vi "FrontPanel.vi"() -> ()   [LabVIEW 2017, in "ImageAcquisitionLibrary.lvlib"]
uses:
  ImageAcquisitionLibrary.lvlib
  StopButton.ctl
  QueueOperations/Message Cluster.ctl
  Acquisition/AcquisitionLoopState.ctl
  Tracking/Tracking State.ctl
  Recording/RecordingState.ctl
  Acquisition/AcquireData.ctl
  MarkersArray.ctl
  Marker.ctl
  <vilib>/Utility/error.llb/DialogType.ctl
  ImageNotifier.vi
  QueueOperations/Enqueue Message (Single).vi
  GlobalFrontPanelReferences.vi
  SettingsGlobal.vi
  MessageQueue.lvlib
panel:
  out "Tracking":i32
  out "Dropped":u32
  out "Image":i32
  in  "Stop":T1
  in  "Settings":bool
  in  "Tracking":bool
  in  "Acquire":bool
  in  "Rec":bool
  out "Image":T2(plugin-control)
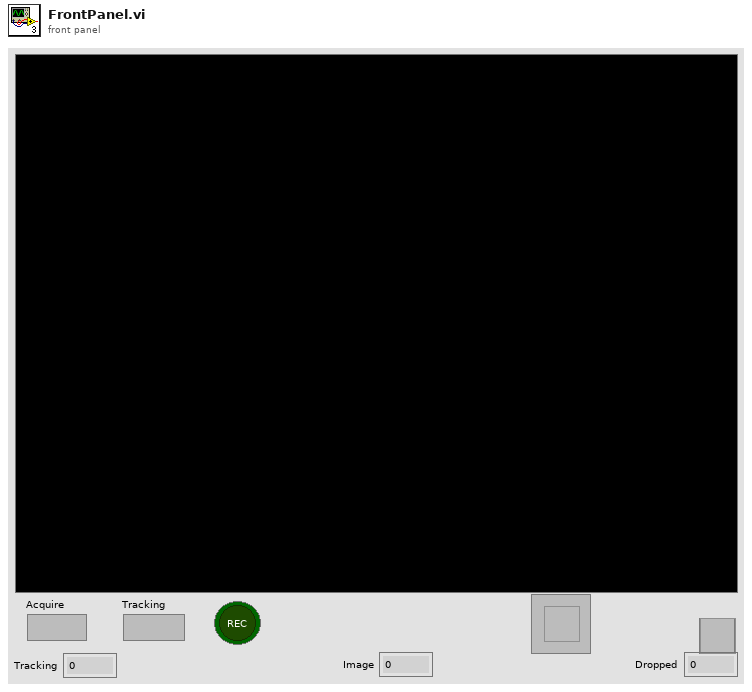
[diagram p1: front panel]
types:
  T1 = typedef "ImageAcquisitionLibrary.lvlib/StopButton.ctl" = bool
  T2 = typedef "IMAQ Image.ctl" = refnum<image>
  T3 = typedef "Image Type" = u32
  T4 = typedef "ImageAcquisitionLibrary.lvlib/AcquireData.ctl" = cluster{"Frame Data":cluster{"Image":u32[][], "Timestamp":timestamp, "Image Type":T3, "Dropped Frames":u32}, "Tracking Data":cluster{"Positions":dbl[][], "Timestamp":timestamp}, "Tracked?":bool}
  T5 = typedef "ImageAcquisitionLibrary.lvlib/RecordingState.ctl" = enum16{"Idle", "Start Recording", "Record", "Update Settings", "Stop Recording", "Exit"}
  T6 = typedef "ImageAcquisitionLibrary.lvlib/Tracking State.ctl" = enum16{"Idle", "Start Tracking", "Track", "Stop Tracking", "Update Settings", "Exit"}
  T7 = typedef "ImageAcquisitionLibrary.lvlib/AcquisitionLoopState.ctl" = enum16{"Start Acquisition", "Acquire", "Stop Acquisition", "Update Settings", "Exit"}
  T8 = typedef "ImageAcquisitionLibrary.lvlib/MessageQueue.lvlib/Message Cluster.ctl" = cluster{"Message":string, "Message Data":variant}
  T9 = typedef "ImageAcquisitionLibrary.lvlib/References.ctl" = cluster{"Acquire":refnum<vi>, "Rec":refnum<vi>, "Tracking":refnum<vi>, "Settings":refnum<vi>, "Stop":refnum<vi>, "Initialized?":bool, "ImDisplay":refnum<vi>}
  T10 = typedef "ImageAcquisitionLibrary.lvlib/Settings.ctl" = cluster{"Harware Configuration":cluster{"Camera":T11, "Frames Per Second":u32, "Simulate Recording":bool, "Simulated Recording Sample":path, "Timestamp Method":enum16{"System Timestamp", "Camera Timestamp", "IMAQdx Timestamp"}}, "Base Recording Path":path, "Type Of Recording":string, "Recording Codec":string, "TrackingSettings":T12, "Calibration":T14, "Broadcast Length":i32}
  T11 = typedef "IMAQdx.ctl" = refnum<k21>
  T12 = typedef "ImageAcquisitionLibrary.lvlib/TrackingSettings.ctl" = cluster{"Max Radius":i32, "Threshold":sgl, "ROI":T13}
  T13 = typedef "IMAQ Rectangle" = cluster{"Left":i32, "Top":i32, "Right":i32, "Bottom":i32, "Rotation":dbl}
  T14 = typedef "ImageAcquisitionLibrary.lvlib/Calibration.ctl" = cluster{"Pixel Width (X)":dbl, "Pixel Height (Y)":dbl}
  T15 = typedef "ImageAcquisitionLibrary.lvlib/MarkersArray.ctl" = T16[]
  T16 = typedef "ImageAcquisitionLibrary.lvlib/Marker.ctl" = cluster{"X":dbl, "Color":u32, "Y ":dbl, "Owner":u8}
  T17 = typedef "DialogType.ctl" = u16
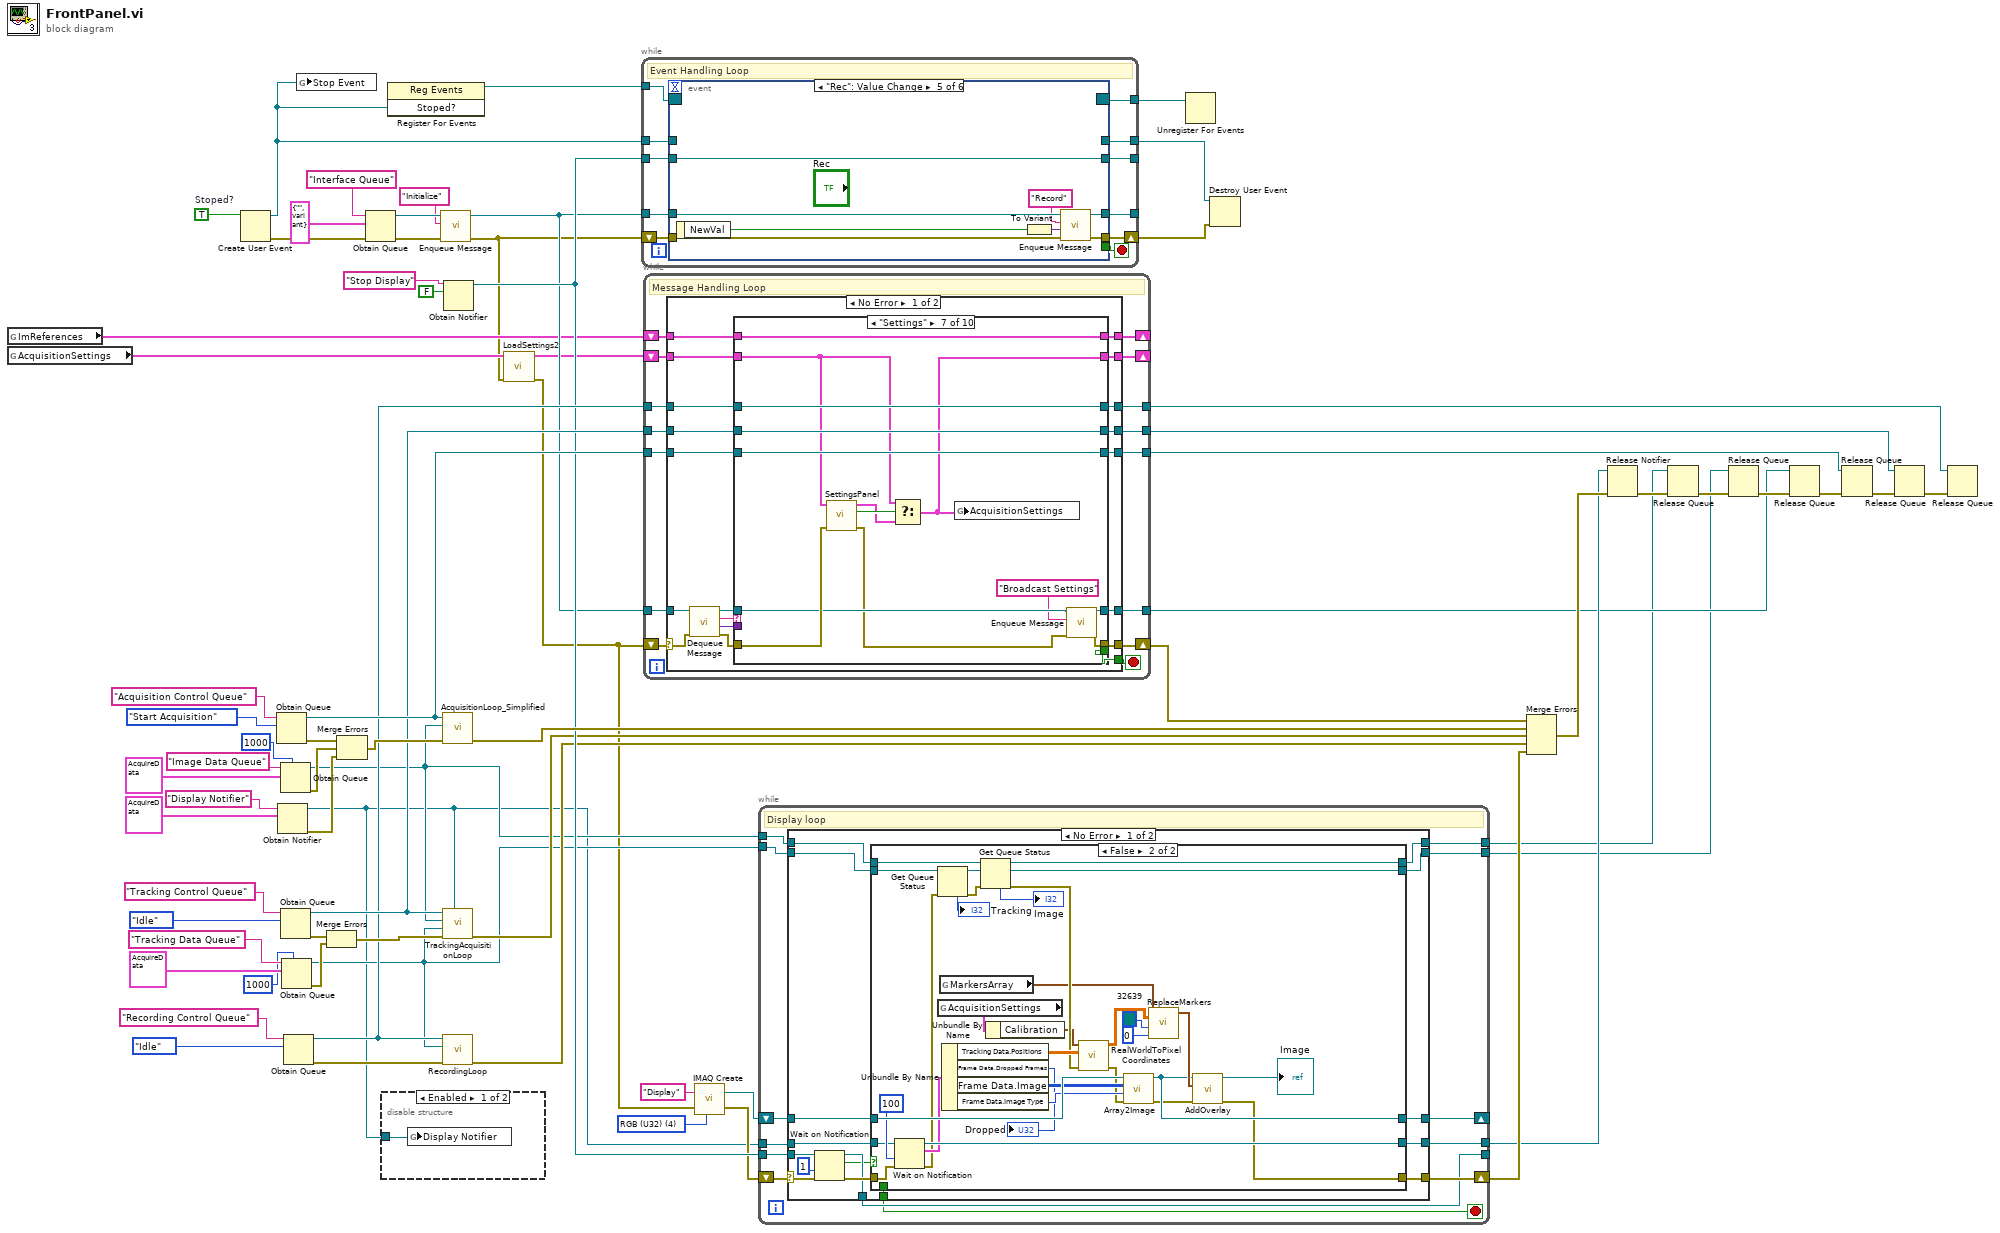
[diagram p0: block diagram]
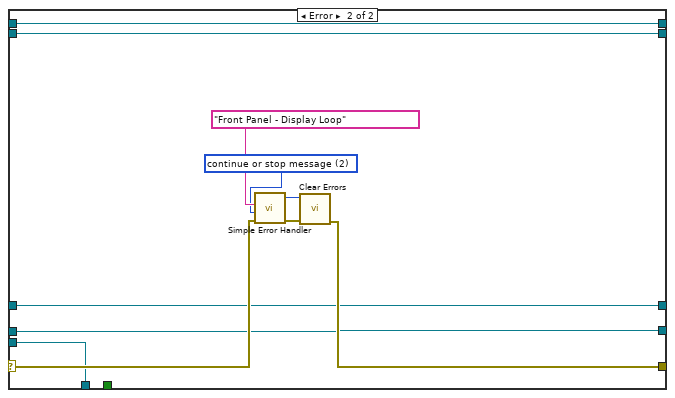
[diagram p4: hidden frame]
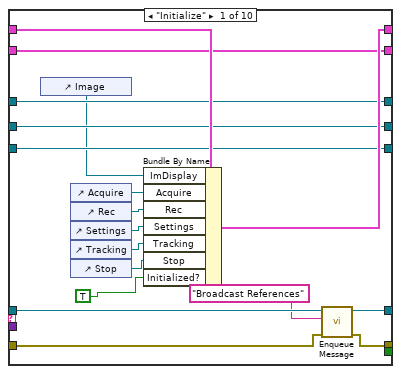
[diagram p5: hidden frame]
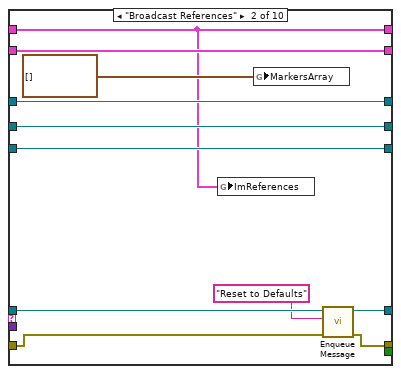
[diagram p6: hidden frame]
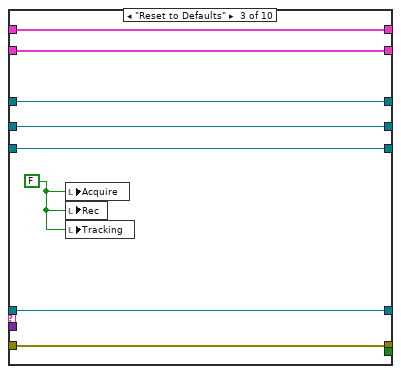
[diagram p7: hidden frame]
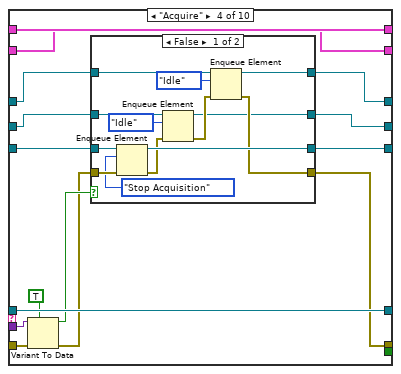
[diagram p8: hidden frame]
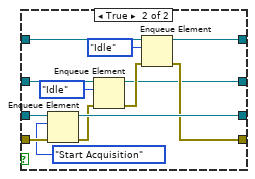
[diagram p9: hidden frame]
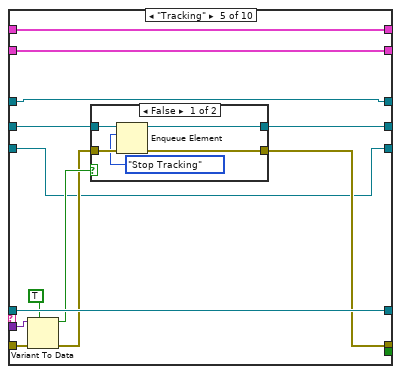
[diagram p10: hidden frame]
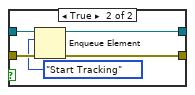
[diagram p11: hidden frame]
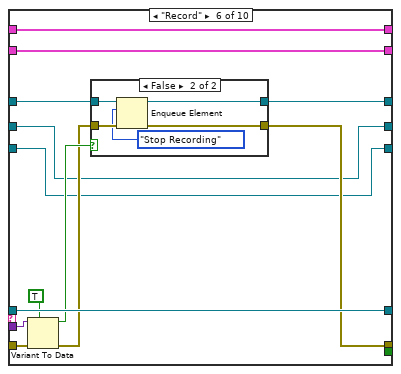
[diagram p12: hidden frame]
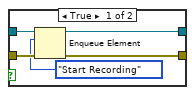
[diagram p13: hidden frame]
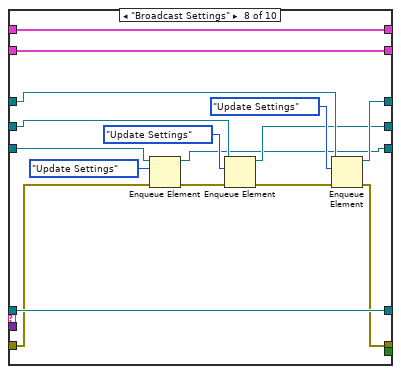
[diagram p14: hidden frame]
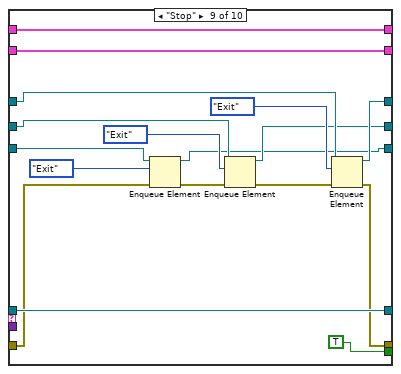
[diagram p15: hidden frame]
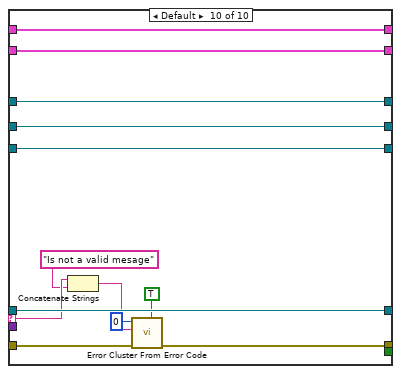
[diagram p16: hidden frame]
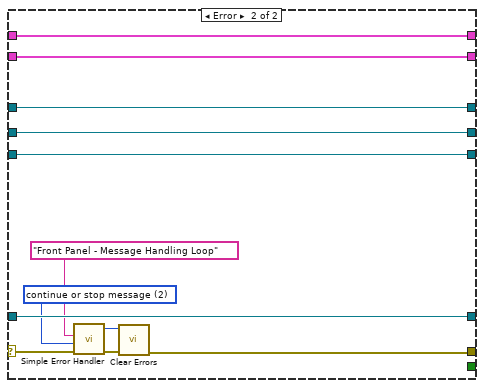
[diagram p17: hidden frame]
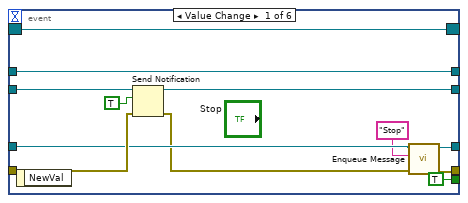
[diagram p18: hidden frame]
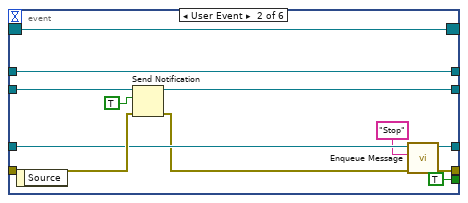
[diagram p19: hidden frame]
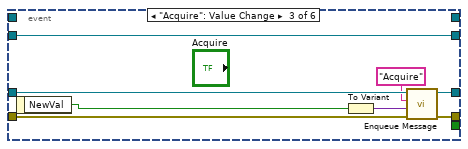
[diagram p20: hidden frame]
diagram:
  w1 = TRUE  # Stoped?
  w34 = T3 4 items=["Grayscale (U8)", "Grayscale (I16)", "Grayscale (SGL)", "Complex (CSG)", "RGB (U32)", "HSL (U32)", "RGB (U64)", "Grayscale (U16)"] ("Image Type")
  n1 = global read "GlobalFrontPanelReferences.vi" "ImReferences"() -> (w10:T9)
  n2 = global read "GlobalFrontPanelReferences.vi" "AcquisitionSettings"() -> (w9:T10)
  n3 = Create User Event(user event datatype=w1) -> (user event=w3:refnum<user-event>, error out=w7:errorcluster)  [unwired: 1 in]
  n4 = Obtain Queue(name (unnamed)="Acquisition Control Queue", element data type=AcquisitionLoopState."Start Acquisition" ("Acquisition State")) -> (queue out=w66:refnum<queue>, error out=w60:errorcluster)  [unwired: 3 in, 1 out]
  n5 = Obtain Notifier(name (unnamed)="Display Notifier", notification data type=T4 {"Frame Data"={"Image"=[], "Timestamp"=timestamp(0 s since 1904-01-01), "Image Type"=0, "Dropped Frames"=0}, "Tracking Data"={"Positions"=[], "Timestamp"=timestamp(0 s since 1904-01-01)}, "Tracked?"=FALSE} ("Acquired Data")) -> (notifier out=w11:refnum<notifier>, error out=w43:errorcluster)  [unwired: 2 in, 1 out]
  n6 = Obtain Queue(max queue size (-1, unlimited)=1000, name (unnamed)="Image Data Queue", element data type=T4 {"Frame Data"={"Image"=[], "Timestamp"=timestamp(0 s since 1904-01-01), "Image Type"=0, "Dropped Frames"=0}, "Tracking Data"={"Positions"=[], "Timestamp"=timestamp(0 s since 1904-01-01)}, "Tracked?"=FALSE} ("Acquired Data")) -> (queue out=w14:refnum<queue>, error out=w58:errorcluster)  [unwired: 2 in, 1 out]
  n7 = Obtain Queue(name (unnamed)="Tracking Control Queue", element data type=Tracking_State."Idle" ("Acquisition State")) -> (queue out=w54:refnum<queue>, error out=w57:errorcluster)  [unwired: 3 in, 1 out]
  n8 = Obtain Queue(max queue size (-1, unlimited)=1000, name (unnamed)="Tracking Data Queue", element data type=T4 {"Frame Data"={"Image"=[], "Timestamp"=timestamp(0 s since 1904-01-01), "Image Type"=0, "Dropped Frames"=0}, "Tracking Data"={"Positions"=[], "Timestamp"=timestamp(0 s since 1904-01-01)}, "Tracked?"=FALSE} ("Acquired Data")) -> (queue out=w23:refnum<queue>, error out=w56:errorcluster)  [unwired: 2 in, 1 out]
  n9 = Obtain Queue(name (unnamed)="Recording Control Queue", element data type=RecordingState."Idle" ("Acquisition State")) -> (queue out=w50:refnum<queue>, error out=w51:errorcluster)  [unwired: 3 in, 1 out]
  n10 = global write "GlobalFrontPanelReferences.vi" "Stop Event"(w3) -> ()
  n11 = Merge Errors(w57, w56) -> (w55:errorcluster)
  n12 = Merge Errors(w60, w58, w43) -> (w59:errorcluster)
  n13 = Obtain Queue(name (unnamed)="Interface Queue", element data type=T8 {"Message"="", "Message Data"=variant} ("Message Cluster"), error in (no error)=w7) -> (queue out=w18:refnum<queue>, error out=w16:errorcluster)  [unwired: 2 in, 1 out]
  n14 = disable-structure shown="Enabled" {
    disable-tunnel: w11 -> [w73 _]
    frame Enabled {
      n15 = global write "ImageNotifier.vi" "Display Notifier"(w73) -> ()
    }
    frame Disabled {
    }
  }
  n16 = register-events(w3) -> (reference out=w6:refnum<event-registration>)  [unwired: 2 in, 1 out]
  n17 = call-poly "Enqueue Message.vi"("error in (no error)"=w16, "Message"="Initialize", "Message Queue"=w18) -> ("error out"=w8:errorcluster, "dup Message Queue"=w17:refnum<queue>)  [unwired: 7 in]
  n18 = call "AcquisitionLoop_Simplified.vi"("error in"=w59, "Image Queue"=w14, "Loop State Queue"=w66) -> ("error out"=w42:errorcluster)  [unwired: 8 in]
  n19 = call "TrackingAcquisitionLoop.vi"("Image Notifier"=w11, "error in (no error)"=w55, "Output Data Queue"=w23, "Input Data Queue"=w14, "Tracking State Queue"=w54) -> ("error out"=w33:errorcluster)  [unwired: 3 in, 3 out]
  n20 = call "RecordingLoop.vi"("error in (no error)"=w51, "Data Queue In"=w23, "State Queue"=w50) -> ("error out"=w32:errorcluster)  [unwired: 7 in, 1 out]
  n21 = Obtain Notifier(name (unnamed)="Stop Display", notification data type=FALSE) -> (notifier out=w37:refnum<notifier>)  [unwired: 2 in, 2 out]
  n22 = call "LoadSettings2.vi"("error in (no error)"=w8, "Settings In"=w9) -> ("error out"=w12:errorcluster, "Settings Out"=w13:T10)  [unwired: 8 in]
  n23 = while {
    tunnel: w17 -> [w84]
    shift-right: [w82] -> w2
    shift-left: w8 -> [w83]
    tunnel: [w81] -> _
    tunnel: w37 -> [w79]
    tunnel: [w78] -> _
    tunnel: w6 -> [w77]
    tunnel: [w76] -> w5
    tunnel: [w75] -> w4
    tunnel: w3 -> [w74]
    stop <- w80 stop-if-true
    # "Event Handling Loop"
    n24 = event shown="[4] \"Rec\": Value Change" {
      selector: w77 -> [w91 w103 _ _ _ _]
      dyn-events: [w91 w103 _ _ _ _] -> w76
      timeout: _ -> [_ _ _ _ _ _]
      tunnel: w84 -> [w89 w100 w113 w118 w128 w136]
      tunnel: w83 -> [w93 w105 w111 w119 w127 w135]
      tunnel: [w87 w98 w110 w120 w130 w134] -> w82
      tunnel: [w88 w101 w112 w121 w129 w137] -> w81
      tunnel: [TRUE TRUE _ _ _ _] -> w80
      tunnel: w79 -> [w95 w107 w115 w123 w131 w138]
      tunnel: [w92 w104 w115 w123 w131 w138] -> w78
      tunnel: [w90 w102 _ _ _ _] -> w75
      tunnel: w74 -> [w90 w102 _ _ _ _]
      event Value Change {
        n25 = event-data() -> ()  [unwired: 1 in, 1 out]
        n26 = Send Notification(notification=TRUE, notifier=w95, error in (no error)=w93) -> (notifier out=w92:refnum<notifier>, error out=w86:errorcluster)
        n27 = call-poly "Enqueue Message.vi"("error in (no error)"=w86, "Message"="Stop", "Message Queue"=w89) -> ("error out"=w87:errorcluster, "dup Message Queue"=w88:refnum<queue>)  [unwired: 7 in]
      }
      event User Event {
        n28 = event-data() -> ()  [unwired: 1 in, 1 out]
        n29 = Send Notification(notification=TRUE, notifier=w107, error in (no error)=w105) -> (notifier out=w104:refnum<notifier>, error out=w99:errorcluster)
        n30 = call-poly "Enqueue Message.vi"("error in (no error)"=w99, "Message"="Stop", "Message Queue"=w100) -> ("error out"=w98:errorcluster, "dup Message Queue"=w101:refnum<queue>)  [unwired: 7 in]
      }
      event "Acquire": Value Change {
        n31 = event-data() -> ("NewVal"=w116:bool)  [unwired: 1 in]
        n32 = To Variant(anything=w116) -> (Variant=w114:variant)
        n33 = call-poly "Enqueue Message.vi"("error in (no error)"=w111, "Message Data"=w114, "Message"="Acquire", "Message Queue"=w113) -> ("error out"=w110:errorcluster, "dup Message Queue"=w112:refnum<queue>)  [unwired: 6 in]
      }
      event "Tracking": Value Change {
        n34 = event-data() -> ("NewVal"=w124:bool)  [unwired: 1 in]
        n35 = To Variant(anything=w124) -> (Variant=w122:variant)
        n36 = call-poly "Enqueue Message.vi"("error in (no error)"=w119, "Message Data"=w122, "Message"="Tracking", "Message Queue"=w118) -> ("error out"=w120:errorcluster, "dup Message Queue"=w121:refnum<queue>)  [unwired: 6 in]
      }
      event "Rec": Value Change {
        n37 = event-data() -> ("NewVal"=w132:bool)  [unwired: 1 in]
        n38 = To Variant(anything=w132) -> (Variant=w126:variant)
        n39 = call-poly "Enqueue Message.vi"("error in (no error)"=w127, "Message Data"=w126, "Message"="Record", "Message Queue"=w128) -> ("error out"=w130:errorcluster, "dup Message Queue"=w129:refnum<queue>)  [unwired: 6 in]
      }
      event "Settings": Value Change {
        n40 = event-data() -> ("NewVal"=w139:bool)  [unwired: 1 in]
        n41 = To Variant(anything=w139) -> ()  [unwired: 1 out]
        n42 = call-poly "Enqueue Message.vi"("error in (no error)"=w135, "Message"="Settings", "Message Queue"=w136) -> ("error out"=w134:errorcluster, "dup Message Queue"=w137:refnum<queue>)  [unwired: 7 in]
      }
    }
  }
  n43 = while {
    shift-right: [w153] -> w69
    shift-left: w12 -> [w154]
    tunnel: w17 -> [w152]
    tunnel: [w151] -> w25
    shift-right: [w148] -> _
    shift-left: w10 -> [w149]
    tunnel: w66 -> [w147]
    tunnel: [w146] -> w24
    tunnel: w54 -> [w145]
    tunnel: [w144] -> w49
    tunnel: w50 -> [w143]
    tunnel: [w142] -> w48
    shift-right: [w140] -> _
    shift-left: w13 -> [w141]
    stop <- w150 stop-if-true
    # "Message Handling Loop"
    n44 = case shown="No Error" w154 {
      selector: w154 -> [w171 w368]
      tunnel: [w173 w364] -> w153
      tunnel: w152 -> [w172 w369]
      tunnel: [w166 w369] -> w151
      tunnel: [w165 _] -> w150
      tunnel: w149 -> [w164 w366]
      tunnel: [w163 w366] -> w148
      tunnel: w147 -> [w162 w361]
      tunnel: [w161 w361] -> w146
      tunnel: w145 -> [w160 w359]
      tunnel: [w159 w359] -> w144
      tunnel: w143 -> [w158 w360]
      tunnel: [w157 w360] -> w142
      tunnel: w141 -> [w156 w358]
      tunnel: [w155 w358] -> w140
      frame No Error {
        n45 = call "Dequeue Message.vi"("error in (no error)"=w171, "Message Queue"=w172) -> ("error out"=w170:errorcluster, "Message Data"=w168:variant, "Message"=w169:string, "dup Message Queue"=w167:refnum<queue>)  [unwired: 6 in]
        n46 = case shown="\"Settings\"" w169 {
          selector: w169 -> [_ _ _ _ _ _ _ _ _ w351]
          tunnel: w170 -> [w176 w196 w210 w222 w261 w284 w307 w316 w333 w349]
          tunnel: [w175 w195 w210 w218 w257 w280 w299 w315 w332 w348] -> w173
          tunnel: w168 -> [_ _ _ w223 w262 w285 _ _ _ _]
          tunnel: w167 -> [w178 w198 w209 w225 w264 w287 w302 w327 w344 w357]
          tunnel: [w177 w197 w209 w225 w264 w287 w301 w327 w344 w357] -> w166
          tunnel: [_ _ _ _ _ _ _ _ TRUE _] -> w165
          tunnel: [w186 w192 w208 w224 w263 w286 w311 w326 w343 w356] -> w163
          tunnel: w164 -> [w191 w192 w208 w224 w263 w286 w311 w326 w343 w356]
          tunnel: w162 -> [w185 w202 w207 w217 w254 w279 w310 w325 w342 w355]
          tunnel: [w185 w202 w207 w216 w254 w279 w310 w313 w330 w355] -> w161
          tunnel: w160 -> [w183 w200 w206 w215 w256 w277 w308 w323 w340 w354]
          tunnel: [w183 w200 w206 w212 w255 w277 w308 w314 w331 w354] -> w159
          tunnel: w158 -> [w184 w201 w205 w214 w253 w278 w309 w320 w337 w353]
          tunnel: [w184 w201 w205 w213 w253 w276 w309 w319 w336 w353] -> w157
          tunnel: w156 -> [w181 w193 w203 w211 w252 w275 w303 w312 w328 w352]
          tunnel: [w181 w193 w203 w211 w252 w275 w304 w312 w328 w352] -> w155
          frame "Initialize" {
            n47 = control-ref of="Image"() -> (w179:refnum<vi>)
            n48 = control-ref of="Acquire"() -> (w190:refnum<vi>)
            n49 = control-ref of="Rec"() -> (w189:refnum<vi>)
            n50 = control-ref of="Settings"() -> (w187:refnum<vi>)
            n51 = control-ref of="Tracking"() -> (w188:refnum<vi>)
            n52 = control-ref of="Stop"() -> (w182:refnum<vi>)
            n53 = Bundle By Name(cluster=w191, "ImDisplay"=w179, "Acquire"=w190, "Rec"=w189, "Settings"=w187, "Tracking"=w188, "Stop"=w182, "Initialized?"=TRUE) -> (w186:T9)
            n54 = call-poly "Enqueue Message.vi"("error in (no error)"=w176, "Message"="Broadcast References", "Message Queue"=w178) -> ("error out"=w175:errorcluster, "dup Message Queue"=w177:refnum<queue>)  [unwired: 7 in]
          }
          frame "Broadcast References" {
            n55 = global write "GlobalFrontPanelReferences.vi" "ImReferences"(w192) -> ()
            n56 = global write "GlobalFrontPanelReferences.vi" "MarkersArray"(T15 [] ("MarkersArray")) -> ()
            n57 = call-poly "Enqueue Message.vi"("error in (no error)"=w196, "Message"="Reset to Defaults", "Message Queue"=w198) -> ("error out"=w195:errorcluster, "dup Message Queue"=w197:refnum<queue>)  [unwired: 7 in]
          }
          frame "Reset to Defaults" {
            w204 = FALSE
            n58 = local write "Acquire"(w204) -> ()
            n59 = local write "Rec"(w204) -> ()
            n60 = local write "Tracking"(w204) -> ()
          }
          frame "Acquire" {
            n61 = Variant To Data(error in=w222, type=TRUE, Variant=w223) -> (data=w220:bool, error out=w219:errorcluster)
            n62 = case shown="False" w220 {
              tunnel: w219 -> [w237 w250]
              tunnel: [w228 w241] -> w218
              tunnel: w217 -> [w235 w248]
              tunnel: [w238 w251] -> w216
              tunnel: w215 -> [w234 w247]
              tunnel: w214 -> [w233 w246]
              tunnel: [w227 w240] -> w213
              tunnel: [w226 w239] -> w212
              frame False {
                n63 = Enqueue Element(queue=w235, element=AcquisitionLoopState."Stop Acquisition" ("Acquisition State"), error in (no error)=w237) -> (queue out=w238:refnum<queue>, error out=w232:errorcluster)  [unwired: 1 in, 1 out]
                n64 = Enqueue Element(queue=w234, element=Tracking_State."Idle", error in (no error)=w232) -> (queue out=w226:refnum<queue>, error out=w229:errorcluster)  [unwired: 1 in, 1 out]
                n65 = Enqueue Element(queue=w233, element=RecordingState."Idle", error in (no error)=w229) -> (queue out=w227:refnum<queue>, error out=w228:errorcluster)  [unwired: 1 in, 1 out]
              }
              frame True {
                n66 = Enqueue Element(queue=w248, element=AcquisitionLoopState."Start Acquisition" ("Acquisition State"), error in (no error)=w250) -> (queue out=w251:refnum<queue>, error out=w245:errorcluster)  [unwired: 1 in, 1 out]
                n67 = Enqueue Element(queue=w247, element=Tracking_State."Idle", error in (no error)=w245) -> (queue out=w239:refnum<queue>, error out=w242:errorcluster)  [unwired: 1 in, 1 out]
                n68 = Enqueue Element(queue=w246, element=RecordingState."Idle", error in (no error)=w242) -> (queue out=w240:refnum<queue>, error out=w241:errorcluster)  [unwired: 1 in, 1 out]
              }
            }
          }
          frame "Tracking" {
            n69 = Variant To Data(error in=w261, type=TRUE, Variant=w262) -> (data=w259:bool, error out=w258:errorcluster)
            n70 = case shown="False" w259 {
              tunnel: w258 -> [w268 w273]
              tunnel: [w267 w272] -> w257
              tunnel: w256 -> [w266 w271]
              tunnel: [w269 w274] -> w255
              frame False {
                n71 = Enqueue Element(queue=w266, element=Tracking_State."Stop Tracking" ("Acquisition State"), error in (no error)=w268) -> (queue out=w269:refnum<queue>, error out=w267:errorcluster)  [unwired: 1 in, 1 out]
              }
              frame True {
                n72 = Enqueue Element(queue=w271, element=Tracking_State."Start Tracking" ("Acquisition State"), error in (no error)=w273) -> (queue out=w274:refnum<queue>, error out=w272:errorcluster)  [unwired: 1 in, 1 out]
              }
            }
          }
          frame "Record" {
            n73 = Variant To Data(error in=w284, type=TRUE, Variant=w285) -> (data=w282:bool, error out=w281:errorcluster)
            n74 = case shown="False" w282 {
              tunnel: w281 -> [w291 w296]
              tunnel: [w290 w295] -> w280
              tunnel: w278 -> [w289 w294]
              tunnel: [w292 w297] -> w276
              frame True {
                n75 = Enqueue Element(queue=w289, element=RecordingState."Start Recording" ("Acquisition State"), error in (no error)=w291) -> (queue out=w292:refnum<queue>, error out=w290:errorcluster)  [unwired: 1 in, 1 out]
              }
              frame False {
                n76 = Enqueue Element(queue=w294, element=RecordingState."Stop Recording" ("Acquisition State"), error in (no error)=w296) -> (queue out=w297:refnum<queue>, error out=w295:errorcluster)  [unwired: 1 in, 1 out]
              }
            }
          }
          frame "Settings" {
            n77 = call "SettingsPanel.vi"("error in"=w307, "Settings In"=w303) -> ("error out"=w300:errorcluster, "Canceled?"=w306:bool, "Settings Out"=w305:T10)  [unwired: 7 in]
            n78 = Select(t=w303, s=w306, f=w305) -> (s? t:f=w304:T10)
            n79 = global write "SettingsGlobal.vi" "AcquisitionSettings"(w304) -> ()
            n80 = call-poly "Enqueue Message.vi"("error in (no error)"=w300, "Message"="Broadcast Settings", "Message Queue"=w302) -> ("error out"=w299:errorcluster, "dup Message Queue"=w301:refnum<queue>)  [unwired: 7 in]
          }
          frame "Broadcast Settings" {
            n81 = Enqueue Element(queue=w325, element=AcquisitionLoopState."Update Settings" ("Acquisition State"), error in (no error)=w316) -> (queue out=w313:refnum<queue>, error out=w321:errorcluster)  [unwired: 1 in, 1 out]
            n82 = Enqueue Element(queue=w323, element=Tracking_State."Update Settings" ("Acquisition State"), error in (no error)=w321) -> (queue out=w314:refnum<queue>, error out=w317:errorcluster)  [unwired: 1 in, 1 out]
            n83 = Enqueue Element(queue=w320, element=RecordingState."Update Settings" ("Acquisition State"), error in (no error)=w317) -> (queue out=w319:refnum<queue>, error out=w315:errorcluster)  [unwired: 1 in, 1 out]
          }
          frame "Stop" {
            n84 = Enqueue Element(queue=w342, element=AcquisitionLoopState."Exit" ("Acquisition State"), error in (no error)=w333) -> (queue out=w330:refnum<queue>, error out=w338:errorcluster)  [unwired: 1 in, 1 out]
            n85 = Enqueue Element(queue=w340, element=Tracking_State."Exit" ("Acquisition State"), error in (no error)=w338) -> (queue out=w331:refnum<queue>, error out=w334:errorcluster)  [unwired: 1 in, 1 out]
            n86 = Enqueue Element(queue=w337, element=RecordingState."Exit" ("Acquisition State"), error in (no error)=w334) -> (queue out=w336:refnum<queue>, error out=w332:errorcluster)  [unwired: 1 in, 1 out]
          }
          frame Default {
            n87 = Concatenate Strings(w351, "Is not a valid mesage" ("error source (\" \")")) -> (w347:string)
            n88 = call <vilib>:"Error Cluster From Error Code.vi"("is warning? (False)"=TRUE, "error in (no error)"=w349, "error message (\"\")"=w347, "error code (0)"=0) -> ("error out"=w348:errorcluster)  [unwired: 5 in]
          }
        }
      }
      frame Error {
        w367 = T17 2 items=["no dialog", "OK message", "continue or stop message", "OK message + warnings", "continue/stop + warnings"] ("type of dialog (OK msg:1)")
        n89 = call <vilib>:"Simple Error Handler.vi"("error source (\" \")"="Front Panel - Message Handling Loop" ("error source (\" \")"), "type of dialog (OK msg:1)"=w367, "error in (no error)"=w368) -> ("code out"=w363:i32, "error out"=w365:errorcluster)  [unwired: 2 in, 3 out]
        n90 = call <vilib>:"Clear Errors.vi"("error in (no error)"=w365, "specific error code to clear (0: all)"=w363) -> ("error out"=w364:errorcluster)  [unwired: 4 in, 1 out]
      }
    }
  }
  n91 = call "IMAQ Create"("Image Name"="Display", "Image Type"=w34, "error in (no error)"=w12) -> ("New Image"=w35:T2, "error out"=w36:errorcluster)  [unwired: 2 in]
  n92 = while {
    tunnel: w11 -> [w372]
    tunnel: w37 -> [w374]
    tunnel: [w381] -> w27
    tunnel: [w375] -> _
    tunnel: w23 -> [w376]
    tunnel: w14 -> [w378]
    tunnel: [w379] -> w22
    tunnel: [w377] -> w21
    shift-right: [w382] -> w28
    shift-left: w36 -> [w373]
    shift-right: [w371] -> _
    shift-left: w35 -> [w380]
    stop <- w370 stop-if-true
    # "Display loop"
    n93 = case shown="No Error" w373 {
      selector: w373 -> [w389 w444]
      tunnel: [w398 w441] -> w382
      tunnel: [w391 w437] -> w381
      tunnel: w380 -> [w397 w436]
      tunnel: [w384 w440] -> w379
      tunnel: w378 -> [w385 w440]
      tunnel: [w383 w439] -> w377
      tunnel: w376 -> [w386 w439]
      tunnel: [w394 w438] -> w375
      tunnel: w374 -> [w392 w438]
      tunnel: w372 -> [w393 w437]
      tunnel: [w390 w436] -> w371
      tunnel: [w387 _] -> w370
      frame No Error {
        n94 = Wait on Notification(notifier=w392, timeout in ms (-1)=1, error in (no error)=w389) -> (notifier out=w394:refnum<notifier>, notification=w388:bool, error out=w396:errorcluster)  [unwired: 1 in, 1 out]
        n95 = case shown="False" w388 {
          selector: w388 -> [w404 _]
          tunnel: [w401 w412] -> w398
          tunnel: w397 -> [w403 w435]
          tunnel: w385 -> [w400 w432]
          tunnel: w386 -> [w399 w431]
          tunnel: w396 -> [w401 w428]
          tunnel: w393 -> [w402 w426]
          tunnel: [w402 w425] -> w391
          tunnel: [w403 w415] -> w390
          tunnel: [w404 _] -> w387
          tunnel: [w400 w422] -> w384
          tunnel: [w399 w421] -> w383
          frame True {
          }
          frame False {
            n96 = Wait on Notification(notifier=w426, timeout in ms (-1)=100, error in (no error)=w428) -> (notifier out=w425:refnum<notifier>, notification=w424:T4, error out=w423:errorcluster)  [unwired: 1 in, 1 out]
            n97 = Get Queue Status(queue=w431, error in (no error)=w423) -> (queue out=w421:refnum<queue>, error out=w430:errorcluster, # elements in queue=→"Tracking":i32)  [unwired: 1 in, 5 out]
            n98 = global read "SettingsGlobal.vi" "AcquisitionSettings"() -> (w409:T10)
            n99 = global read "GlobalFrontPanelReferences.vi" "MarkersArray"() -> (w405:T15)
            n100 = Unbundle By Name(w424) -> ("Tracking Data.Positions"=w411:dbl[][], "Frame Data.Dropped Frames"=→"Dropped":u32, "Frame Data.Image"=w434:u32[][], "Frame Data.Image Type"=w433:T3)
            n101 = Get Queue Status(queue=w432, error in (no error)=w430) -> (queue out=w422:refnum<queue>, error out=w410:errorcluster, # elements in queue=→"Image":i32)  [unwired: 1 in, 5 out]
            n102 = Unbundle By Name(w409) -> ("Calibration"=w408:T14)
            n103 = call "RealWorldToPixelCoordinates.vi"("error in (no error)"=w410, "Real World Points"=w411, "Calibration 2"=w408) -> ("error out"=w406:errorcluster, "Pixels"=w407:dbl[][])  [unwired: 6 in]
            n104 = call "Array2Image.vi"("error in (no error)"=w406, "Image Type"=w433, "Image Pixels (U32)"=w434, "Image 2"=w435) -> ("error out"=w413:errorcluster, "Image"=w415:T2)  [unwired: 6 in]
            n105 = call "ReplaceMarkers.vi"("Owner"=u8 0, "Color"=u32 32639, "Pixels 3"=w407, "MarkersArray"=w405) -> ("MarkersArray Out"=w416:T15)  [unwired: 6 in, 1 out]
            n106 = call "AddOverlay.vi"("error in (no error)"=w413, "MarkersArray"=w416, "Refnum in"=w415) -> ("error out"=w412:errorcluster, "Refnum out"=→"Image":T2)  [unwired: 7 in]
          }
        }
      }
      frame Error {
        w442 = T17 2 items=["no dialog", "OK message", "continue or stop message", "OK message + warnings", "continue/stop + warnings"] ("type of dialog (OK msg:1)")
        n107 = call <vilib>:"Simple Error Handler.vi"("error source (\" \")"="Front Panel - Display Loop" ("error source (\" \")"), "type of dialog (OK msg:1)"=w442, "error in (no error)"=w444) -> ("code out"=w445:i32, "error out"=w443:errorcluster)  [unwired: 2 in, 3 out]
        n108 = call <vilib>:"Clear Errors.vi"("error in (no error)"=w443, "specific error code to clear (0: all)"=w445) -> ("error out"=w441:errorcluster)  [unwired: 4 in, 1 out]
      }
    }
  }
  n109 = Unregister For Events(event registration refnum=w5) -> ()  [unwired: 1 in, 1 out]
  n110 = Destroy User Event(user event=w4, error in=w2) -> ()  [unwired: 1 out]
  n111 = Merge Errors(w69, w42, w33, w32, w28) -> (w29:errorcluster)
  n112 = Release Notifier(notifier=w27, error in (no error)=w29) -> (error out=w26:errorcluster)  [unwired: 1 in, 2 out]
  n113 = Release Queue(queue=w22, error in (no error)=w26) -> (error out=w30:errorcluster)  [unwired: 1 in, 2 out]
  n114 = Release Queue(queue=w21, error in (no error)=w30) -> (error out=w31:errorcluster)  [unwired: 1 in, 2 out]
  n115 = Release Queue(queue=w25, error in (no error)=w31) -> (error out=w39:errorcluster)  [unwired: 1 in, 2 out]
  n116 = Release Queue(queue=w24, error in (no error)=w39) -> (error out=w47:errorcluster)  [unwired: 1 in, 2 out]
  n117 = Release Queue(queue=w49, error in (no error)=w47) -> (error out=w46:errorcluster)  [unwired: 1 in, 2 out]
  n118 = Release Queue(queue=w48, error in (no error)=w46) -> ()  [unwired: 1 in, 3 out]
